vi "irmonitor.vi"() -> ()   [LabVIEW 2014]
uses:
  <vilib>/Utility/file.llb/Read From Spreadsheet File (string).vi
panel:
  out "Temperature against Time":cluster{timestamp[], dbl[]}[](graph)
  out "new picture":picture caption="Temperature against Humidity"
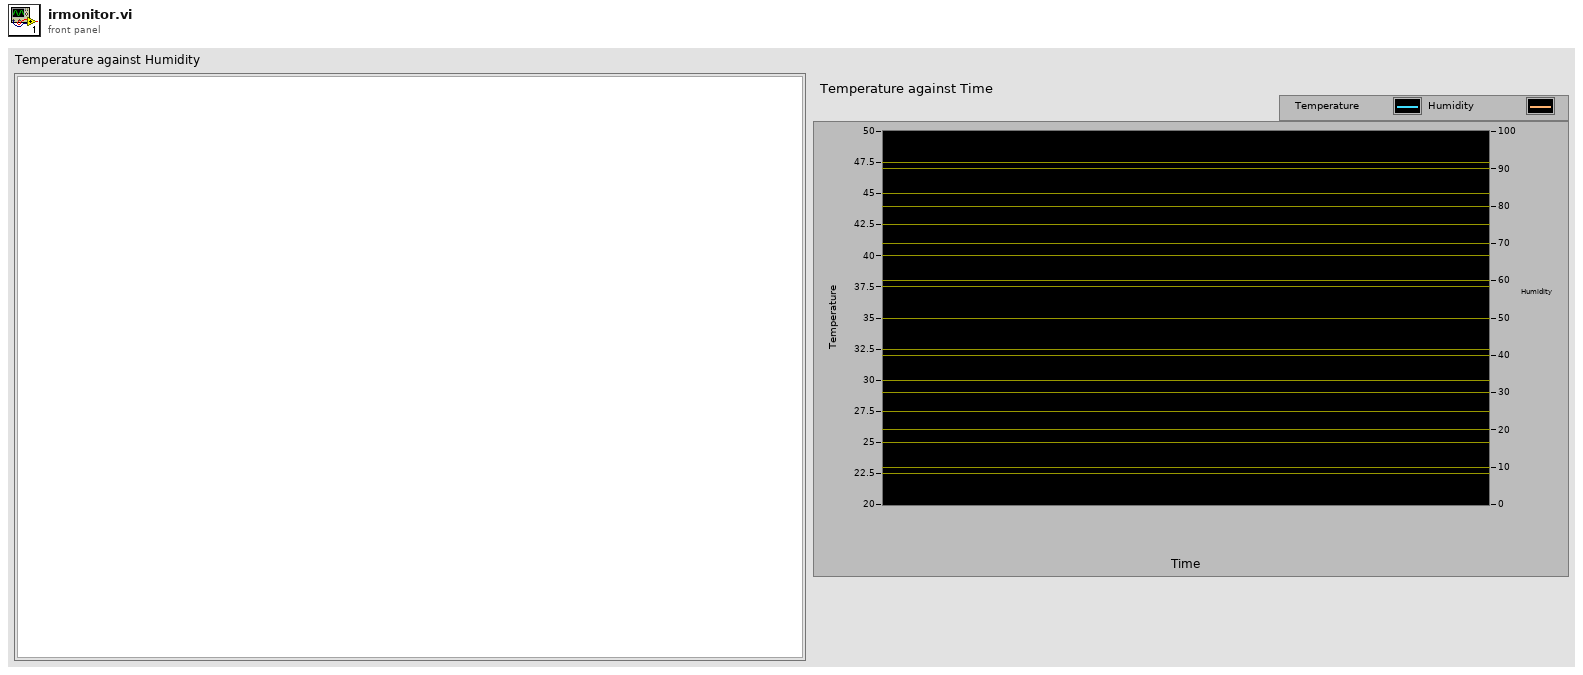
[diagram p1: front panel]
types:
  T1 = typedef "imagedata.ctl" = cluster{"image type":i32, "image depth":i32, "image":u8[], "mask":u8[], "colors":u32[], "Rectangle":cluster{"left":i16, "top":i16, "right":i16, "bottom":i16}}
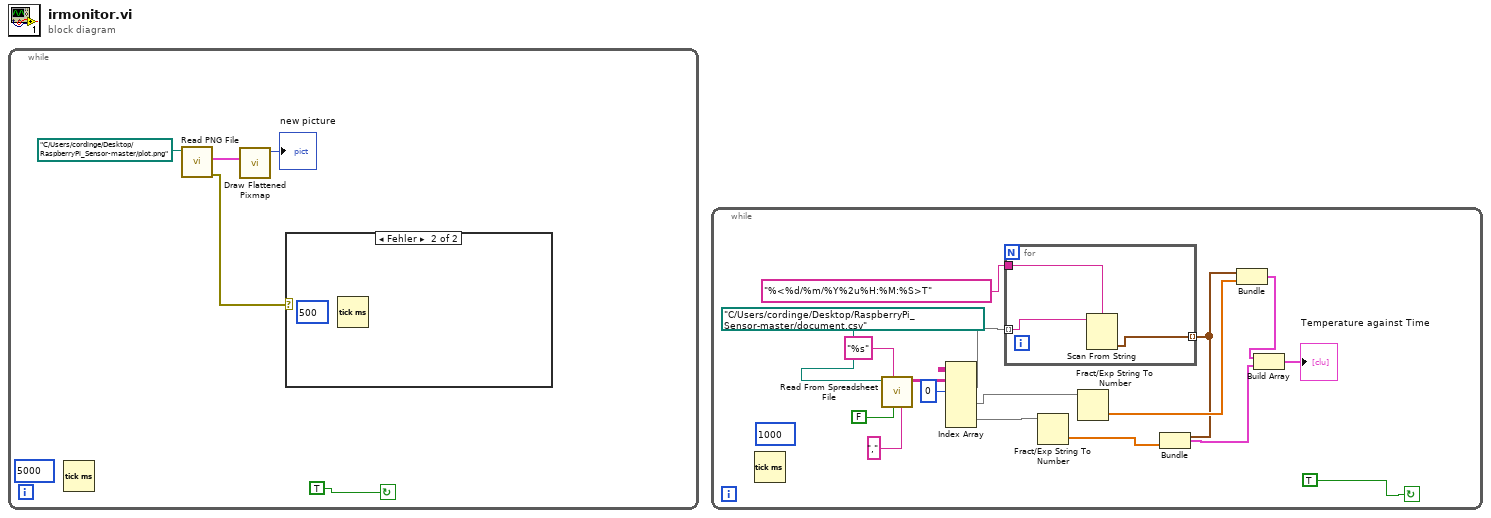
[diagram p0: block diagram]
diagram:
  n1 = while {
    stop <- TRUE continue-if-true
    (unwired) u32 5000 ("Timer-Wert (ms)")
    n2 = Tick Count (ms)() -> ()  [unwired: 1 out]
    n3 = call <vilib>:"Read PNG File.vi"("path to PNG file"=path "C:/Users/cordinge/Desktop/RaspberryPi_Sensor-master/plot.png") -> ("error out"=w1:errorcluster, "image data"=w4:T1)  [unwired: 8 in, 1 out]
    n4 = call <vilib>:"Draw Flattened Pixmap.vi"("image data"=w4) -> ("new picture"=→"new picture":picture)  [unwired: 8 in]
    n5 = case shown="Fehler" w1 {
      frame No Error {
      }
      frame Error {
        (unwired) u32 500 ("Timer-Wert (ms)")
        n6 = Tick Count (ms)() -> ()  [unwired: 1 out]
      }
    }
  }
  n7 = while {
    stop <- TRUE continue-if-true
    (unwired) u32 1000 ("Timer-Wert (ms)")
    n8 = Tick Count (ms)() -> ()  [unwired: 1 out]
    n9 = call-poly <vilib>:"Read From Spreadsheet File.vi"("delimiter (\\t)"="," ("delimiter (\\t)"), "transpose (no:F)"=FALSE, "format (%s)"="%s", "file path (dialog if empty)"=path "C:/Users/cordinge/Desktop/RaspberryPi_Sensor-master/document.csv") -> ("all rows"=w22:string[][])  [unwired: 3 in, 4 out]
    n10 = Index Array(array=w22, index (col) #1=0 ("Deaktivierter Index (Spalte)")) -> (element #1=w20:string[], element #2=w18:string[], element #3=w15:string[])  [unwired: 5 in]
    n11 = for {
      tunnel: w20 -> [w25] mode=indexing
      tunnel: "%<%d/%m/%Y%2u%H:%M:%S>T" ("Format-String") -> [w24]
      tunnel: [w23] -> w16 mode=indexing
      n12 = Scan From String(format string=w24, input string=w25) -> (output 1=w23:timestamp)  [unwired: 3 in, 3 out]
    }
    n13 = Fract/Exp String To Number(string=w15) -> (number=w14:dbl[])  [unwired: 3 in, 1 out]
    n14 = Fract/Exp String To Number(string=w18) -> (number=w17:dbl[])  [unwired: 3 in, 1 out]
    n15 = Bundle(w16, w14) -> (w8:cluster{timestamp[], dbl[]})  [unwired: 1 in]
    n16 = Bundle(w16, w17) -> (w9:cluster{timestamp[], dbl[]})  [unwired: 1 in]
    n17 = Build Array(w9, w8) -> (→"Temperature against Time":cluster{timestamp[], dbl[]}[])
  }
